vi "Render.vi"(7 "Data":refnum<class "Datum.lvclass">, 8 "Error In":errorcluster, 10 "Abstract Syntax Tree":refnum<class "Root.lvclass">, 11 "Compiler In":refnum<class "Compiler.lvclass">) -> (0 "Error Out":errorcluster, 2 "Writer":refnum<class "Writer.lvclass">, 3 "Compiler Out":refnum<class "Compiler.lvclass">)   [LabVIEW 2018, in "Toolkit.lvlib" / "Compiler.lvclass"]
uses:
  Compiler.lvclass
  Writers/Writer/Writer.lvclass
  Nodes/Root/Root.lvclass
  Data/Datum/Datum.lvclass
  Compiler.lvclass/Compiler.ctl
  Renderer/Renderer.lvclass
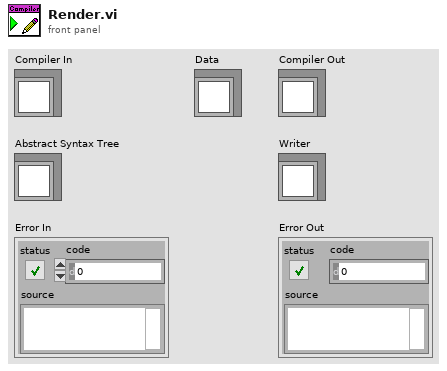
[diagram p1: front panel]
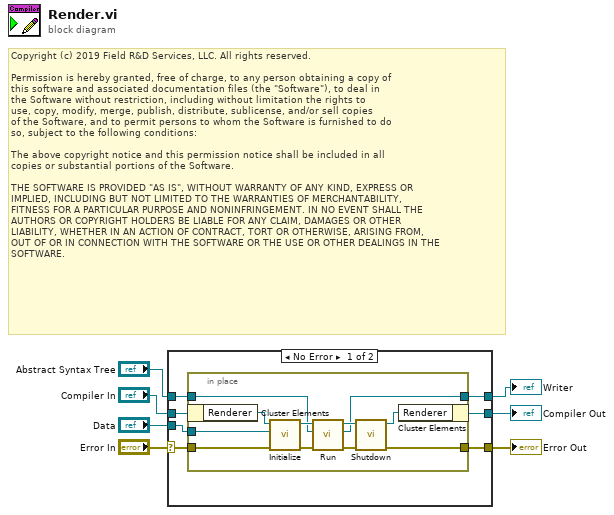
[diagram p0: block diagram]
diagram:
  # "Copyright (c) 2019 Field R&D Services, LLC. All rights reserved.\n\nPermission is hereby granted, free of charge, to any person obtaining a copy of\nthis software and associated documentation files (the \"Software\"), to deal in\nthe Software without restriction, including without limitation the rights to\nuse, copy, modify, merge, publish, distribute, sublicense, and/or sell copies\nof the Software, and to permit persons to whom the Software is furnished to do\nso, subject to the following conditions:\n\nThe above copyright notice and this permission notice shall be included in all\ncopies or substantial portions of the Software.\n\nTHE SOFTWARE IS PROVIDED \"AS IS\", WITHOUT WARRANTY OF ANY KIND, EXPRESS OR\nIMPLIED, INCLUDING BUT NOT LIMITED TO THE WARRANTIES OF MERCHANTABILITY,\nFITNESS FOR A PARTICULAR PURPOSE AND NONINFRINGEMENT. IN NO EVENT SHALL THE\nAUTHORS OR COPYRIGHT HOLDERS BE LIABLE FOR ANY CLAIM, DAMAGES OR OTHER\nLIABILITY, WHETHER IN AN ACTION OF CONTRACT, TORT OR OTHERWISE, ARISING FROM,\nOUT OF OR IN CONNECTION WITH THE SOFTWARE OR THE USE OR OTHER DEALINGS IN THE\nSOFTWARE."
  n1 = case shown="No Error" "Error In" {
    selector: "Error In" -> [w13 w27]
    tunnel: [w11 w27] -> w6
    tunnel: "Compiler In" -> [w14 w26]
    tunnel: [w12 w26] -> w4
    tunnel: [w10 _] -> w3
    tunnel: "Abstract Syntax Tree" -> [w9 _]
    tunnel: "Data" -> [w8 _]
    frame No Error {
      n2 = in-place {
        in-place-border: w13 -> [w24]
        in-place-border: [w25] -> w11
        in-place-border: [w18] -> w10
        in-place-border: w9 -> [w16]
        in-place-border: w8 -> [w15]
        n3 = in-place-cluster #1(w14) -> ("Renderer"=w23:refnum<class "Renderer.lvclass">)
        n4 = call-dynamic "Initialize.vi"("Error In"=w24, "Data"=w15, "Renderer In"=w23) -> ("Error Out"=w19:errorcluster, "Renderer Out"=w21:refnum<class "Renderer.lvclass">)  [unwired: 7 in]
        n5 = call-dynamic "Run.vi"("Error In"=w19, "Abstract Syntax Tree"=w16, "Renderer In"=w21) -> ("Error Out"=w17:errorcluster, "Writer"=w18:refnum<class "Writer.lvclass">, "Renderer Out"=w20:refnum<class "Renderer.lvclass">)  [unwired: 6 in]
        n6 = call-dynamic "Shutdown.vi"("Error In"=w17, "Renderer In"=w20) -> ("Error Out"=w25:errorcluster, "Renderer Out"=w22:refnum<class "Renderer.lvclass">)  [unwired: 7 in, 1 out]
        n7 = in-place-cluster #1("Renderer"=w22) -> (w12:refnum<class "Compiler.lvclass">)
      }
    }
    frame Error {
    }
  }
  "Error Out" <- w6
  "Compiler Out" <- w4
  "Writer" <- w3
